vi "List to comma string.vi"(11 "Array":string[](array[string])) -> (3 "String":string)   [LabVIEW 2015, in "SLSC Switch.lvclass"]
uses:
  SLSC Switch.lvclass
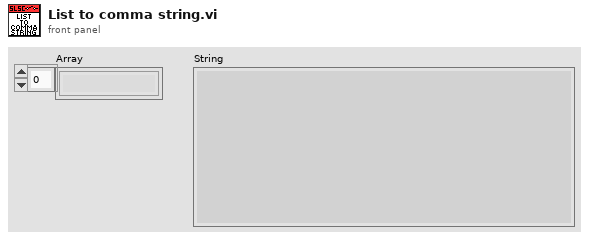
[diagram p1: front panel]
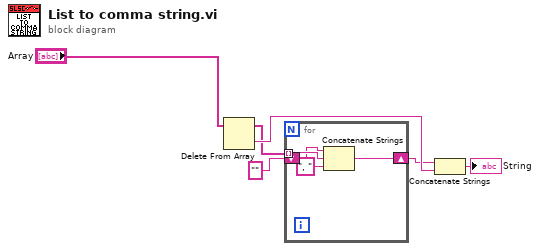
[diagram p0: block diagram]
diagram:
  n1 = Delete From Array(array="Array") -> (deleted portion=w5:string, array with subset deleted=w2:string[])  [unwired: 2 in]
  n2 = for {
    tunnel: w2 -> [w9] mode=indexing
    shift-right: [w7] -> w4
    shift-left: "" ("string") -> [w8]
    n3 = Concatenate Strings(w8, w9, ", " ("string")) -> (w7:string)
  }
  n4 = Concatenate Strings(w4, w5) -> (→"String":string)
